vi "getTaskReference.vi"(8 "error in (no error)":errorcluster, 11 "ITask in":refnum<class "ITask.lvclass">) -> (0 "error out":errorcluster, 2 "taskRef":refnum<vi>, 3 "ITask out":refnum<class "ITask.lvclass">)   [LabVIEW 2023, in "TLC_Daemon.lvlib" / "ITask.lvclass"]
doc: "Returns the VI reference related to the task to handle."
uses:
  ITask.lvclass
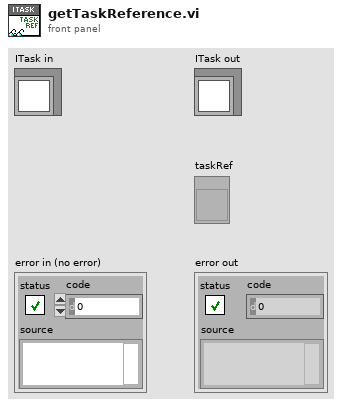
[diagram p1: front panel]
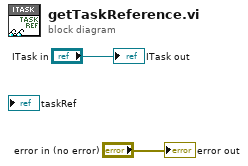
[diagram p0: block diagram]
diagram:
  "error out" <- "error in (no error)"
  "ITask out" <- "ITask in"
